vi "ReadTrajectory_JSON_FIle_WriteGlobal_Example.vi"() -> ()   [LabVIEW 2019]
uses:
  SubVI/read_json_StoreTrajectory_GlobalVariable.vi
panel:
  out "error out":errorcluster
  # "Read Trajectory JSON File and \nWrite to Global Variable"
  # "See block diagram"
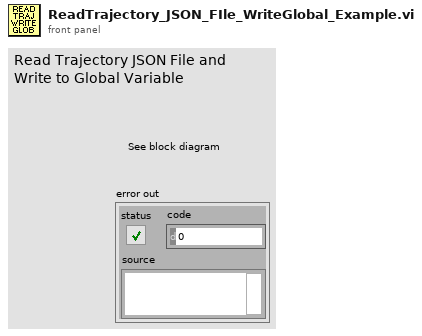
[diagram p1: front panel]
types:
  T1 = typedef "Trajectory_Library.lvlib/TRAJECTORY.ctl" = cluster{"TotalTImeSecs":dbl, "States":T2[]}
  T2 = typedef "Trajectory_Library.lvlib/TRAJ_STATE.ctl" = cluster{"TimeSeconds":dbl, "Velocity":dbl, "Acceleration":dbl, "POSE":T3, "Curvature":dbl}
  T3 = typedef "Trajectory_Library.lvlib/POSE2D.ctl" = cluster{"TRANSLATION":T4, "ROTATION":T5}
  T4 = typedef "Trajectory_Library.lvlib/TRANSLATION2D.ctl" = cluster{"X":dbl, "Y":dbl}
  T5 = typedef "Trajectory_Library.lvlib/ROTATION2D.ctl" = cluster{"VALUE":dbl, "COS":dbl, "SIN":dbl}
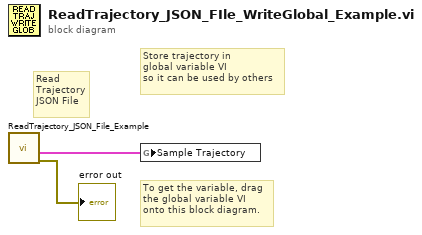
[diagram p0: block diagram]
diagram:
  # "To get the variable, drag\nthe global variable VI\nonto this block diagram."
  # "Read\nTrajectory\nJSON File"
  # "Store trajectory in\nglobal variable VI\nso it can be used by others"
  n1 = call "ReadTrajectory_JSON_File_Example.vi"() -> ("error out"=→"error out":errorcluster, "outTRAJECTORY"=w2:T1)  [unwired: 8 in, 2 out]
  n2 = global write "read_json_StoreTrajectory_GlobalVariable.vi" "Sample Trajectory"(w2) -> ()
